vi "Leitura.vi"() -> ()   [LabVIEW 2018]
uses:
  <vilib>/Instr/_visa.llb/VISA Configure Serial Port (Instr).vi
panel:
  in  "Conectar":bool
  in  "Combo Box 4":string(combo)
  in  "Combo Box 3":string(combo)
  in  "Combo Box 2":string(combo)
  in  "Combo Box":string(combo)
  out "Umidade 4":bool
  out "Umidade 3":bool
  out "Umidade 2":bool
  out "Leitura do sensor 4":dbl
  out "Leitura do sensor 3":dbl
  out "Leitura do sensor 2":dbl
  in  "Sensor 4":bool
  in  "Sensor 3":bool
  in  "Sensor 2":bool
  in  "Sensor 1":bool
  out "Saida de erro":T1
  in  "Salvar arquivo de sinal em:":path
  out "Umidade":bool
  in  "Limite inferior de umidade":dbl
  in  "Limite superior de umidade":dbl
  out "Waveform Chart":T2(graph)
  out "Leitura do sensor":dbl
  in  "Parar leituras":bool
  in  "Porta de leitura do sensor de umidade":refnum<visa-resource-name>
  # "Porta de comunicações"
  # "Sensores do sistema"
  # "Leitura do sensor 1"
  # "Leitura do sensor 2"
  # "Leitura do sensor 3"
  # "Leitura do sensor 4"
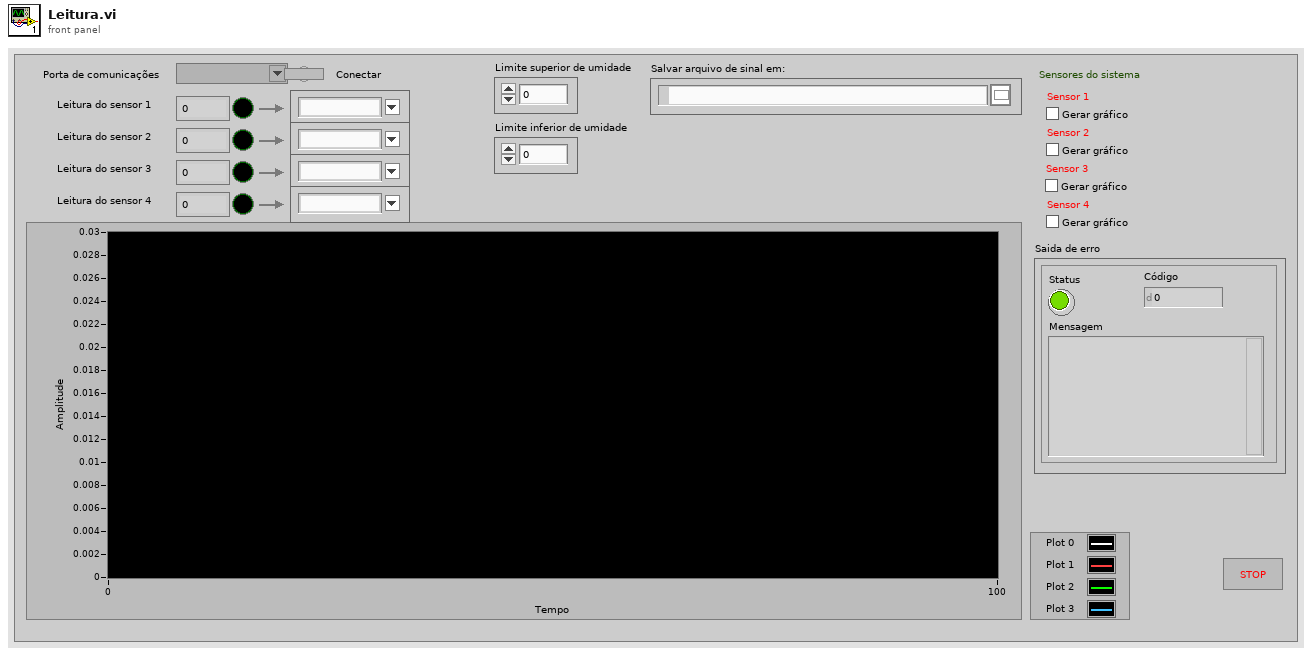
[diagram p1: front panel]
types:
  T1 = cluster{"Status":bool, "Código":i32, "Mensagem":string}
  T2 = cluster{"[0]":dbl, "[1]":dbl, "[2]":dbl, "[3]":dbl}
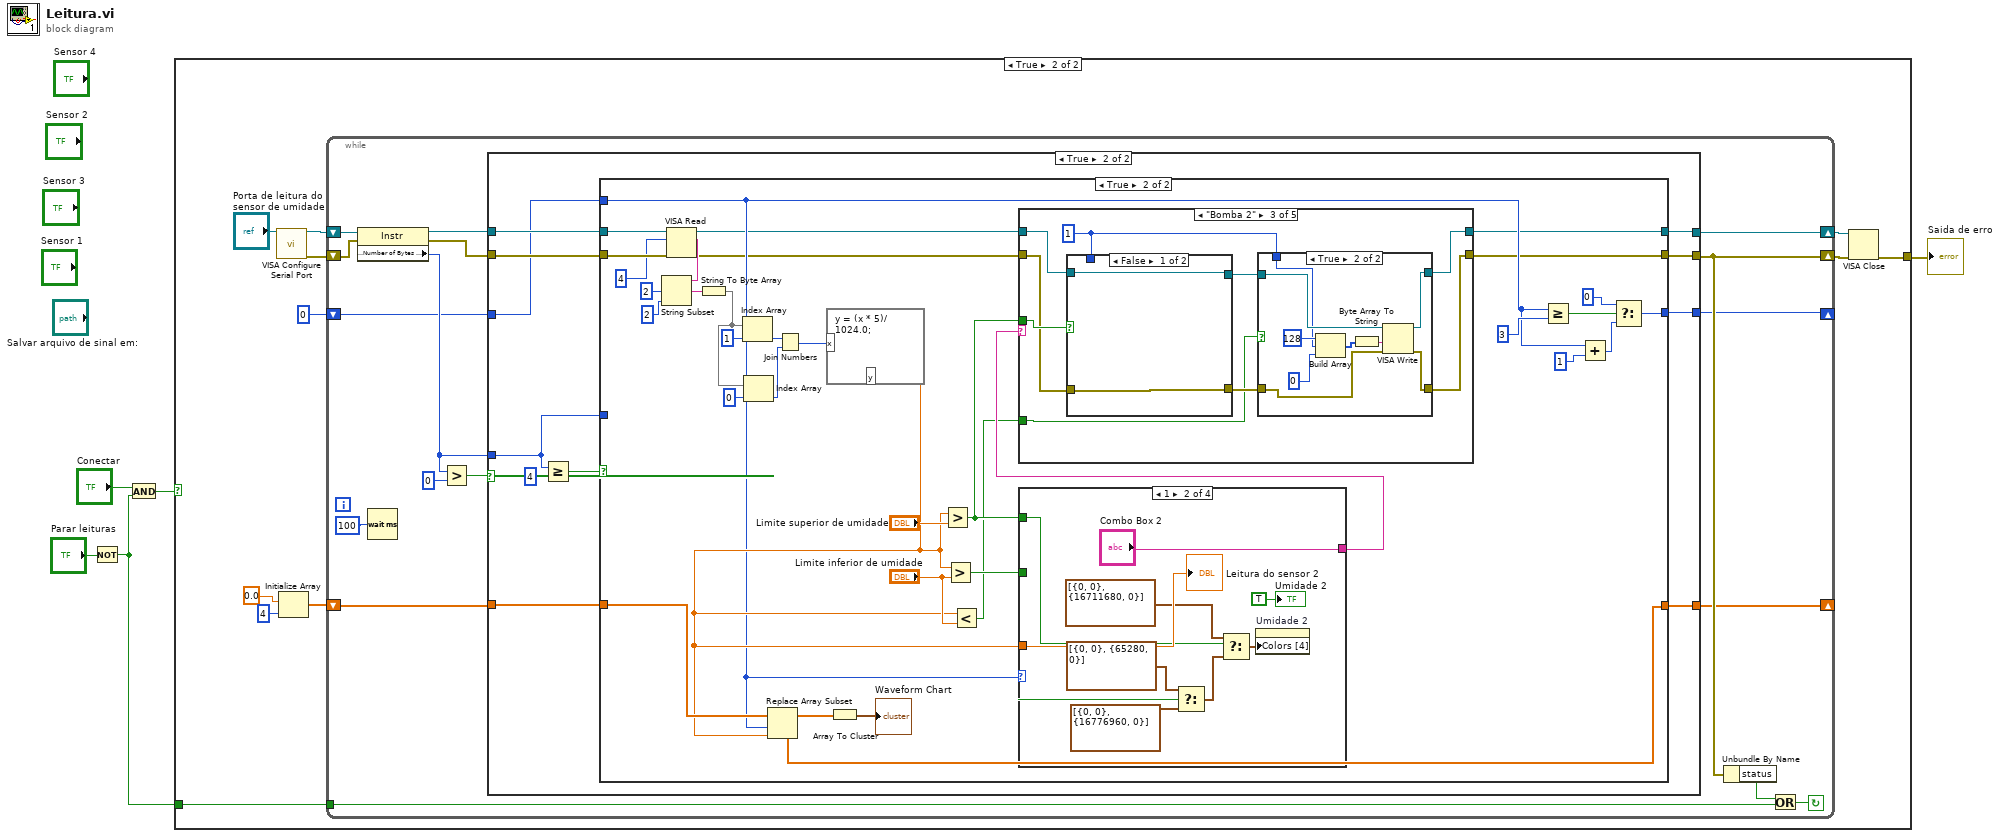
[diagram p0: block diagram]
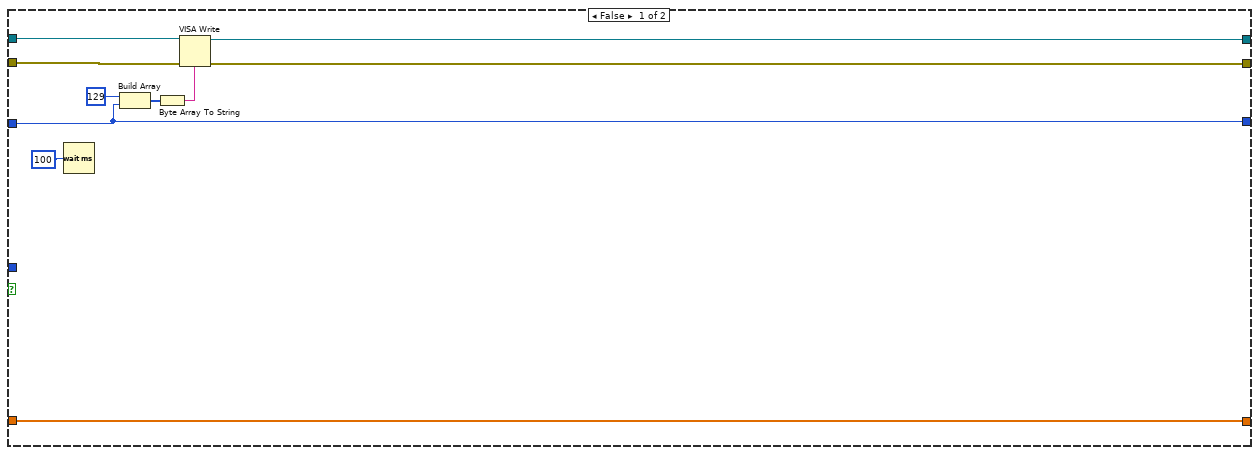
[diagram p3: hidden frame]
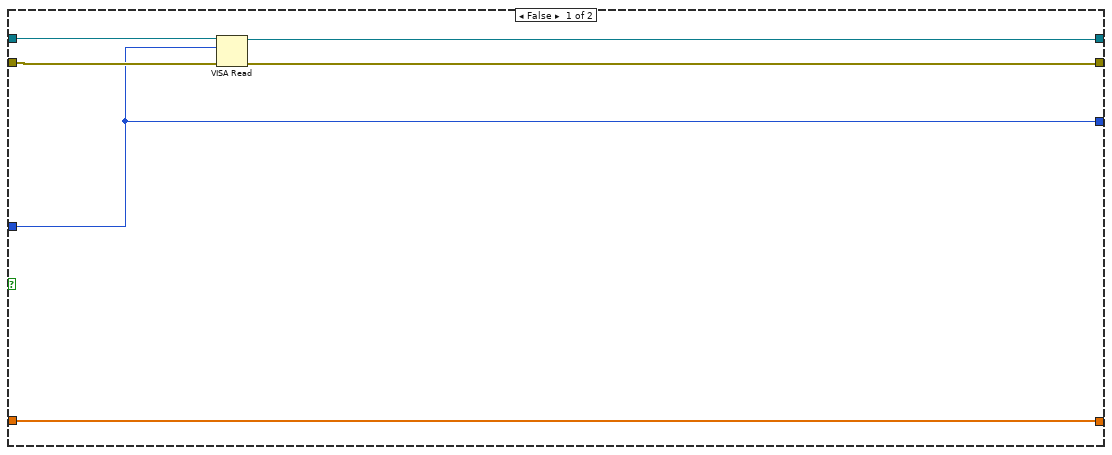
[diagram p4: hidden frame]
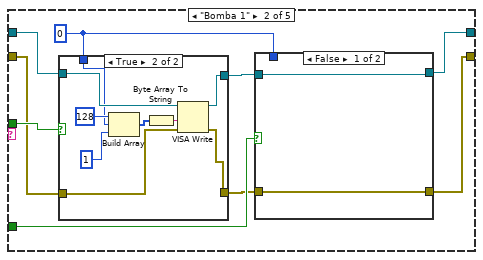
[diagram p6: hidden frame]
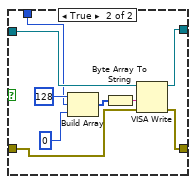
[diagram p7: hidden frame]
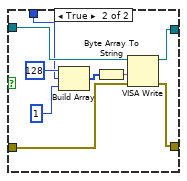
[diagram p10: hidden frame]
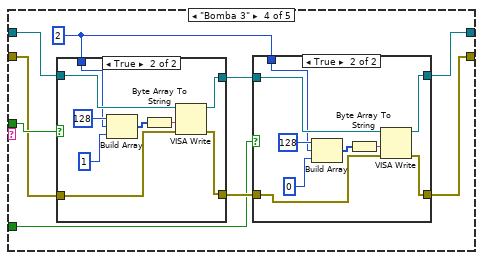
[diagram p11: hidden frame]
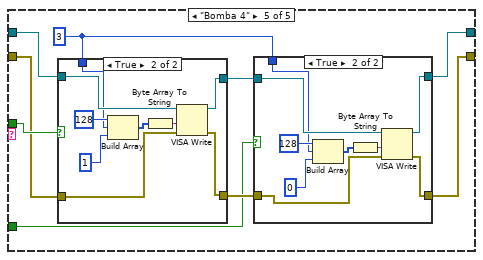
[diagram p14: hidden frame]
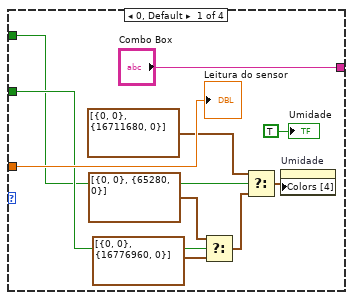
[diagram p17: hidden frame]
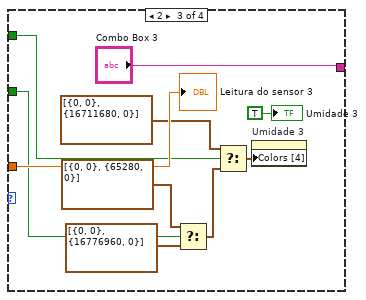
[diagram p18: hidden frame]
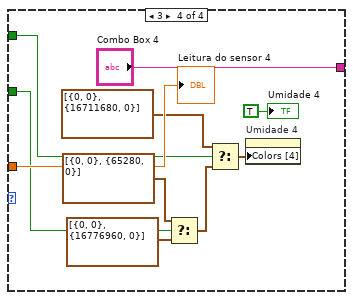
[diagram p19: hidden frame]
diagram:
  n1 = Not(x="Parar leituras") -> (.not. x?=w2:bool)
  n2 = And(x="Conectar", y=w2) -> (x .and. y?=w5:bool)
  n3 = case shown="True" w5 {
    tunnel: w2 -> [_ w15]
    tunnel: [_ w14] -> w1
    frame False {
    }
    frame True {
      n4 = call-poly "VISA Configure Serial Port"("VISA resource name"="Porta de leitura do sensor de umidade") -> ("VISA resource name out"=w13:refnum<visa-resource-name>, "error out"=w11:errorcluster)  [unwired: 13 in]
      n5 = Initialize Array(0.0 ("element"), 4 ("dimension size")) -> (w6:dbl[])
      n6 = while {
        tunnel: w15 -> [w28]
        shift-right: [w23] -> w12
        shift-left: w13 -> [w27]
        shift-right: [w22] -> w10
        shift-left: w11 -> [w26]
        shift-right: [w19] -> _
        shift-left: 0 -> [w20]
        shift-right: [w17] -> _
        shift-left: w6 -> [w18]
        stop <- w30 continue-if-true
        n7 = property class="Instr"(reference=w27, error in=w26) -> (reference out=w25:refnum<visa-resource-name>, error out=w24:errorcluster, "Serial Settings:Number of Bytes at Serial Port"=w21:u32)
        n8 = Wait (ms)(milliseconds to wait=u32 100) -> ()  [unwired: 1 out]
        n9 = Greater?(x=w21, y=u32 0) -> (0:w31:bool)
        n10 = case shown="True" w31 {
          tunnel: w25 -> [w40 w52]
          tunnel: w24 -> [w39 w51]
          tunnel: [w38 w50] -> w23
          tunnel: [w37 w49] -> w22
          tunnel: w21 -> [_ w47]
          tunnel: w20 -> [w35 w48]
          tunnel: [w35 w46] -> w19
          tunnel: w18 -> [w34 w45]
          tunnel: [w34 w44] -> w17
          frame False {
            n11 = Wait (ms)(milliseconds to wait=u32 100) -> ()  [unwired: 1 out]
            n12 = Build Array(u8 129 ("element"), w35) -> (w42:u32[])
            n13 = Byte Array To String(unsigned byte array=w42) -> (string=w41:string)
            n14 = VISA Write(VISA resource name=w40, write buffer=w41, error in (no error)=w39) -> (VISA resource name out=w38:refnum<visa-resource-name>, error out=w37:errorcluster)  [unwired: 1 out]
          }
          frame True {
            n15 = Greater Or Equal?(x=w47, y=u32 4) -> (x >= y?=w53:bool)
            n16 = case shown="True" w53 {
              tunnel: w52 -> [w60 w92]
              tunnel: w51 -> [w59 w91]
              tunnel: [w58 w62] -> w50
              tunnel: [w57 w61] -> w49
              tunnel: w48 -> [_ w67]
              tunnel: w47 -> [w56 _]
              tunnel: [w56 w74] -> w46
              tunnel: w45 -> [w55 w72]
              tunnel: [w55 w69] -> w44
              frame False {
                n17 = VISA Read(VISA resource name=w60, byte count=w56, error in (no error)=w59) -> (VISA resource name out=w58:refnum<visa-resource-name>, error out=w57:errorcluster)  [unwired: 2 out]
              }
              frame True {
                n18 = VISA Read(VISA resource name=w92, byte count=u32 4, error in (no error)=w91) -> (VISA resource name out=w65:refnum<visa-resource-name>, read buffer=w89:string, error out=w64:errorcluster)  [unwired: 1 out]
                n19 = String Subset(string=w89, offset (0)=2, length (rest)=2 ("length (rest)")) -> (substring=w87:string)
                n20 = String To Byte Array(string=w87) -> (unsigned byte array=w84:u8[])
                n21 = Index Array(array=w84, index=1) -> (element=w83:u8)
                n22 = Index Array(array=w84, index=0) -> (element=w82:u8)
                n23 = Join Numbers(hi=w83, lo=w82) -> ((hi.lo)=w81:u16)
                n24 = formula code="y = (x * 5)/1024.0;"("x"=w81) -> ("y"=w71:dbl)
                n25 = Replace Array Subset(array=w72, new element=w71, index=w67) -> (w69:dbl[])
                n26 = Array To Cluster(array=w69) -> (cluster=→"Waveform Chart":T2)
                n27 = Greater?(x=w71, y="Limite superior de umidade") -> (0:w66:bool)
                n28 = Greater?(x=w71, y="Limite inferior de umidade") -> (0:w73:bool)
                n29 = Less?(x=w71, y="Limite inferior de umidade") -> (x < y?=w63:bool)
                n30 = case shown="1" w67 {
                  tunnel: w71 -> [w230 w240 w250 w260]
                  tunnel: w73 -> [w226 w232 w242 w252]
                  tunnel: w66 -> [w224 w233 w243 w253]
                  tunnel: ["Combo Box" "Combo Box 2" "Combo Box 3" "Combo Box 4"] -> w68
                  frame 0, Default {
                    n31 = Select(t=cluster{u32, u32}[] [{0, 0}, {65280, 0}] ("Colors [4]"), s=w226, f=cluster{u32, u32}[] [{0, 0}, {16776960, 0}] ("Colors [4]")) -> (s? t:f=w228:cluster{u32, u32}[])
                    n32 = Select(t=cluster{u32, u32}[] [{0, 0}, {16711680, 0}] ("Colors [4]"), s=w224, f=w228) -> (s? t:f=w229:cluster{u32, u32}[])
                    n33 = property on="Umidade" class="Bool (strict)"("Colors [4]"=w229) -> ()  [unwired: 2 in, 2 out]
                    "Leitura do sensor" <- w230
                    "Umidade" <- TRUE ("Boolean")
                  }
                  frame 1 {
                    n34 = Select(t=cluster{u32, u32}[] [{0, 0}, {65280, 0}] ("Colors [4]"), s=w232, f=cluster{u32, u32}[] [{0, 0}, {16776960, 0}] ("Colors [4]")) -> (s? t:f=w239:cluster{u32, u32}[])
                    n35 = Select(t=cluster{u32, u32}[] [{0, 0}, {16711680, 0}] ("Colors [4]"), s=w233, f=w239) -> (s? t:f=w234:cluster{u32, u32}[])
                    n36 = property on="Umidade 2" class="Bool (strict)"("Colors [4]"=w234) -> ()  [unwired: 2 in, 2 out]
                    "Leitura do sensor 2" <- w240
                    "Umidade 2" <- TRUE ("Umidade 2")
                  }
                  frame 2 {
                    n37 = Select(t=cluster{u32, u32}[] [{0, 0}, {65280, 0}] ("Colors [4]"), s=w242, f=cluster{u32, u32}[] [{0, 0}, {16776960, 0}] ("Colors [4]")) -> (s? t:f=w249:cluster{u32, u32}[])
                    n38 = Select(t=cluster{u32, u32}[] [{0, 0}, {16711680, 0}] ("Colors [4]"), s=w243, f=w249) -> (s? t:f=w244:cluster{u32, u32}[])
                    n39 = property on="Umidade 3" class="Bool (strict)"("Colors [4]"=w244) -> ()  [unwired: 2 in, 2 out]
                    "Leitura do sensor 3" <- w250
                    "Umidade 3" <- TRUE ("Umidade 3")
                  }
                  frame 3 {
                    n40 = Select(t=cluster{u32, u32}[] [{0, 0}, {65280, 0}] ("Colors [4]"), s=w252, f=cluster{u32, u32}[] [{0, 0}, {16776960, 0}] ("Colors [4]")) -> (s? t:f=w259:cluster{u32, u32}[])
                    n41 = Select(t=cluster{u32, u32}[] [{0, 0}, {16711680, 0}] ("Colors [4]"), s=w253, f=w259) -> (s? t:f=w254:cluster{u32, u32}[])
                    n42 = property on="Umidade 4" class="Bool (strict)"("Colors [4]"=w254) -> ()  [unwired: 2 in, 2 out]
                    "Leitura do sensor 4" <- w260
                    "Umidade 4" <- TRUE ("Umidade 4")
                  }
                }
                n43 = case shown="\"Bomba 2\"" w68 {
                  tunnel: w66 -> [_ w105 w132 w163 w194]
                  tunnel: w65 -> [w95 w104 w131 w161 w192]
                  tunnel: w64 -> [w96 w103 w130 w162 w193]
                  tunnel: w63 -> [_ w102 w133 w164 w195]
                  tunnel: [w95 w101 w128 w159 w190] -> w62
                  tunnel: [w96 w100 w129 w160 w191] -> w61
                  frame "Nenhuma", Default {
                  }
                  frame "Bomba 1" {
                    w97 = u8 0 ("element")
                    n44 = case shown="True" w105 {
                      tunnel: w104 -> [w118 w124]
                      tunnel: [w118 w123] -> w99
                      tunnel: w103 -> [w117 w122]
                      tunnel: [w117 w121] -> w98
                      tunnel: w97 -> [_ w119]
                      frame False {
                      }
                      frame True {
                        n45 = Build Array(u8 128 ("element"), w119, u8 1 ("element")) -> (w126:u8[])
                        n46 = Byte Array To String(unsigned byte array=w126) -> (string=w125:string)
                        n47 = VISA Write(VISA resource name=w124, write buffer=w125, error in (no error)=w122) -> (VISA resource name out=w123:refnum<visa-resource-name>, error out=w121:errorcluster)  [unwired: 1 out]
                      }
                    }
                    n48 = case shown="False" w102 {
                      tunnel: w99 -> [w107 w112]
                      tunnel: [w107 w111] -> w101
                      tunnel: w98 -> [w106 w110]
                      tunnel: [w106 w109] -> w100
                      tunnel: w97 -> [_ w108]
                      frame False {
                      }
                      frame True {
                        n49 = Build Array(u8 128 ("element"), w108, u8 0 ("element")) -> (w115:u8[])
                        n50 = Byte Array To String(unsigned byte array=w115) -> (string=w114:string)
                        n51 = VISA Write(VISA resource name=w112, write buffer=w114, error in (no error)=w110) -> (VISA resource name out=w111:refnum<visa-resource-name>, error out=w109:errorcluster)  [unwired: 1 out]
                      }
                    }
                  }
                  frame "Bomba 2" {
                    w134 = u8 1 ("element")
                    n52 = case shown="False" w132 {
                      tunnel: w131 -> [w149 w155]
                      tunnel: [w149 w154] -> w136
                      tunnel: w130 -> [w148 w153]
                      tunnel: [w148 w152] -> w135
                      tunnel: w134 -> [_ w150]
                      frame False {
                      }
                      frame True {
                        n53 = Build Array(u8 128 ("element"), w150, u8 1 ("element")) -> (w157:u8[])
                        n54 = Byte Array To String(unsigned byte array=w157) -> (string=w156:string)
                        n55 = VISA Write(VISA resource name=w155, write buffer=w156, error in (no error)=w153) -> (VISA resource name out=w154:refnum<visa-resource-name>, error out=w152:errorcluster)  [unwired: 1 out]
                      }
                    }
                    n56 = case shown="True" w133 {
                      tunnel: w136 -> [w138 w143]
                      tunnel: [w138 w142] -> w128
                      tunnel: w135 -> [w137 w141]
                      tunnel: [w137 w140] -> w129
                      tunnel: w134 -> [_ w139]
                      frame False {
                      }
                      frame True {
                        n57 = Build Array(u8 128 ("element"), w139, u8 0 ("element")) -> (w146:u8[])
                        n58 = Byte Array To String(unsigned byte array=w146) -> (string=w145:string)
                        n59 = VISA Write(VISA resource name=w143, write buffer=w145, error in (no error)=w141) -> (VISA resource name out=w142:refnum<visa-resource-name>, error out=w140:errorcluster)  [unwired: 1 out]
                      }
                    }
                  }
                  frame "Bomba 3" {
                    w165 = u8 2 ("element")
                    n60 = case shown="True" w163 {
                      tunnel: w161 -> [w180 w186]
                      tunnel: [w180 w185] -> w167
                      tunnel: w162 -> [w179 w184]
                      tunnel: [w179 w183] -> w166
                      tunnel: w165 -> [_ w181]
                      frame False {
                      }
                      frame True {
                        n61 = Build Array(u8 128 ("element"), w181, u8 1 ("element")) -> (w188:u8[])
                        n62 = Byte Array To String(unsigned byte array=w188) -> (string=w187:string)
                        n63 = VISA Write(VISA resource name=w186, write buffer=w187, error in (no error)=w184) -> (VISA resource name out=w185:refnum<visa-resource-name>, error out=w183:errorcluster)  [unwired: 1 out]
                      }
                    }
                    n64 = case shown="True" w164 {
                      tunnel: w167 -> [w169 w174]
                      tunnel: [w169 w173] -> w159
                      tunnel: w166 -> [w168 w172]
                      tunnel: [w168 w171] -> w160
                      tunnel: w165 -> [_ w170]
                      frame False {
                      }
                      frame True {
                        n65 = Build Array(u8 128 ("element"), w170, u8 0 ("element")) -> (w177:u8[])
                        n66 = Byte Array To String(unsigned byte array=w177) -> (string=w176:string)
                        n67 = VISA Write(VISA resource name=w174, write buffer=w176, error in (no error)=w172) -> (VISA resource name out=w173:refnum<visa-resource-name>, error out=w171:errorcluster)  [unwired: 1 out]
                      }
                    }
                  }
                  frame "Bomba 4" {
                    w196 = u8 3 ("element")
                    n68 = case shown="True" w194 {
                      tunnel: w192 -> [w211 w217]
                      tunnel: [w211 w216] -> w198
                      tunnel: w193 -> [w210 w215]
                      tunnel: [w210 w214] -> w197
                      tunnel: w196 -> [_ w212]
                      frame False {
                      }
                      frame True {
                        n69 = Build Array(u8 128 ("element"), w212, u8 1 ("element")) -> (w219:u8[])
                        n70 = Byte Array To String(unsigned byte array=w219) -> (string=w218:string)
                        n71 = VISA Write(VISA resource name=w217, write buffer=w218, error in (no error)=w215) -> (VISA resource name out=w216:refnum<visa-resource-name>, error out=w214:errorcluster)  [unwired: 1 out]
                      }
                    }
                    n72 = case shown="True" w195 {
                      tunnel: w198 -> [w200 w205]
                      tunnel: [w200 w204] -> w190
                      tunnel: w197 -> [w199 w203]
                      tunnel: [w199 w202] -> w191
                      tunnel: w196 -> [_ w201]
                      frame False {
                      }
                      frame True {
                        n73 = Build Array(u8 128 ("element"), w201, u8 0 ("element")) -> (w208:u8[])
                        n74 = Byte Array To String(unsigned byte array=w208) -> (string=w207:string)
                        n75 = VISA Write(VISA resource name=w205, write buffer=w207, error in (no error)=w203) -> (VISA resource name out=w204:refnum<visa-resource-name>, error out=w202:errorcluster)  [unwired: 1 out]
                      }
                    }
                  }
                }
                n76 = Greater Or Equal?(x=w67, y=3) -> (x >= y?=w78:bool)
                n77 = Add(x=w67, y=1) -> (x+y=w75:u32)
                n78 = Select(t=0, s=w78, f=w75) -> (s? t:f=w74:u32)
              }
            }
          }
        }
        n79 = Unbundle By Name(w22) -> ("status"=w29:bool)
        n80 = Or(x=w29, y=w28) -> (x .or. y?=w30:bool)
      }
      n81 = VISA Close(VISA resource name=w12, error in (no error)=w10) -> (error out=w14:errorcluster)
    }
  }
  "Saida de erro" <- w1
